vi "Expand.vi"(8 "error in (no error)":errorcluster, 11 "CollapsePanel in":refnum<class "CollapsePanel.lvclass">) -> (0 "error out":errorcluster, 3 "CollapsePanel out":refnum<class "CollapsePanel.lvclass">)   [LabVIEW 2021, in "CollapsePanel.lvclass"]
uses:
  CollapsePanel.lvclass
  CollapsePanel.lvclass/CollapsePanel.ctl
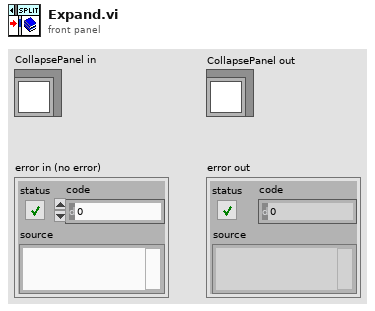
[diagram p1: front panel]
types:
  T1 = enum16{"No Scaling", "Scale All Objects", "Scale Single Object"}
  T2 = typedef "CollapsePanel.lvclass/collapse direction.ctl" = enum16{"Left", "Right", "Up", "Down"}
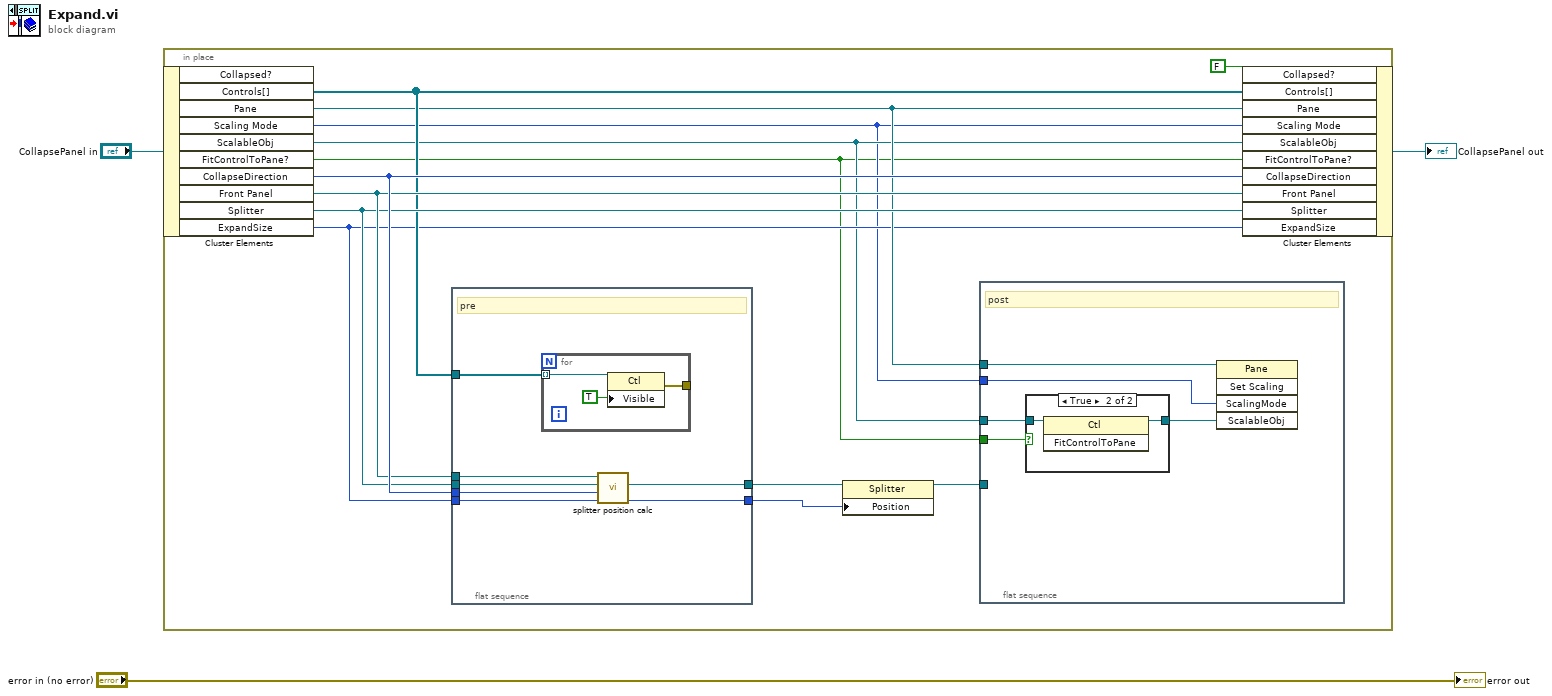
[diagram p0: block diagram]
diagram:
  n1 = in-place {
    n2 = in-place-cluster #1("CollapsePanel in") -> ("Controls[]"=w12:refnum<vi>[], "Pane"=w11:refnum<vi>, "Scaling Mode"=w8:T1, "ScalableObj"=w9:refnum<vi>, "FitControlToPane?"=w7:bool, "CollapseDirection"=w15:T2, "Front Panel"=w14:refnum<vi>, "Splitter"=w13:refnum<vi>, "ExpandSize"=w10:i32)  [unwired: 1 out]
    n3 = flat-sequence {
      tunnel: [w25] -> w16
      tunnel: w15 -> [w26]
      tunnel: w14 -> [w28]
      tunnel: w13 -> [w29]
      tunnel: w12 -> [w31]
      tunnel: w10 -> [w27]
      tunnel: [w30] -> w6
      frame #0 {
        # "pre"
        n4 = for {
          tunnel: w31 -> [w33] mode=indexing
          tunnel: [w32] -> _
          n5 = property on="Property Node" class="Ctl"(reference=w33, "Visible"=TRUE) -> (error out=w32:errorcluster)  [unwired: 1 in, 1 out]
        }
        n6 = call "splitter position calc.vi"("ExpandSize"=w27, "CollapseDirection"=w26, "Splitter"=w29, "Front Panel"=w28) -> ("Splitter Position"=w25:i32, "Splitter"=w30:refnum<vi>)  [unwired: 5 in, 1 out]
      }
    }
    n7 = property class="Splitter"(reference=w6, "Position"=w16) -> (reference out=w5:refnum<vi>)  [unwired: 1 in, 1 out]
    n8 = flat-sequence {
      tunnel: w11 -> [w20]
      tunnel: w9 -> [w19]
      tunnel: w8 -> [w18]
      tunnel: w7 -> [w17]
      tunnel: w5 -> [_]
      frame #0 {
        # "post"
        n9 = case shown="True" w17 {
          tunnel: w19 -> [w22 w24]
          tunnel: [w22 w23] -> w21
          frame False {
          }
          frame True {
            n10 = invoke class="Ctl" method="FitControlToPane"(reference=w24) -> (reference out=w23:refnum<vi>)  [unwired: 2 in, 2 out]
          }
        }
        n11 = invoke class="Pane" method="Set Scaling"(reference=w20, "ScalingMode"=w18, "ScalableObj"=w21) -> ()  [unwired: 2 in, 5 out]
      }
    }
    n12 = in-place-cluster #1("Collapsed?"=FALSE, "Controls[]"=w12, "Pane"=w11, "Scaling Mode"=w8, "ScalableObj"=w9, "FitControlToPane?"=w7, "CollapseDirection"=w15, "Front Panel"=w14, "Splitter"=w13, "ExpandSize"=w10) -> (→"CollapsePanel out":refnum<class "CollapsePanel.lvclass">)
  }
  "error out" <- "error in (no error)"
